vi "add_PointStamped.vi"(5 "Point":cluster{"x":dbl, "y":dbl, "z":dbl}, 6 "Stamp":cluster{"frame_id":string, "reset seq?":bool}, 7 "msg in":string) -> (3 "msg out":string)   [LabVIEW 2016]
doc: "Flattens a point stamped into a message"
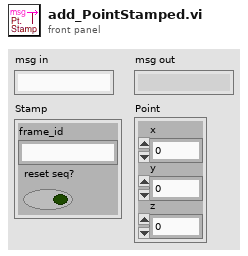
[diagram p1: front panel]
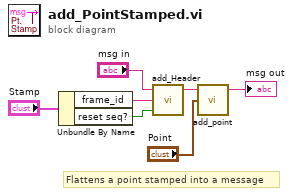
[diagram p0: block diagram]
diagram:
  # "Flattens a point stamped into a message"
  n1 = Unbundle By Name("Stamp") -> ("frame_id"=w2:string, "reset seq?"=w1:bool)
  n2 = call "add_Header.vi"("reset seq?"=w1, "frame_id"=w2, "msg in"="msg in") -> ("msg out"=w5:string)  [unwired: 2 in]
  n3 = call "add_point.vi"("Point"="Point", "msg in"=w5) -> ("msg out"=→"msg out":string)  [unwired: 3 in]
